vi "CRYMain Menu Process LIB LIB.vi"(9 "sOption":string, 11 "sAction":string) -> (2 "sData_Out":string)   [LabVIEW 2013]
uses:
  CRYProject/CRYProject Editor Global.vi
  CRYMainGlobal.vi
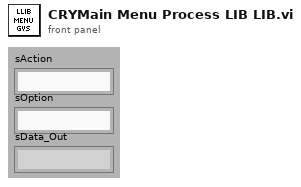
[diagram p1: front panel]
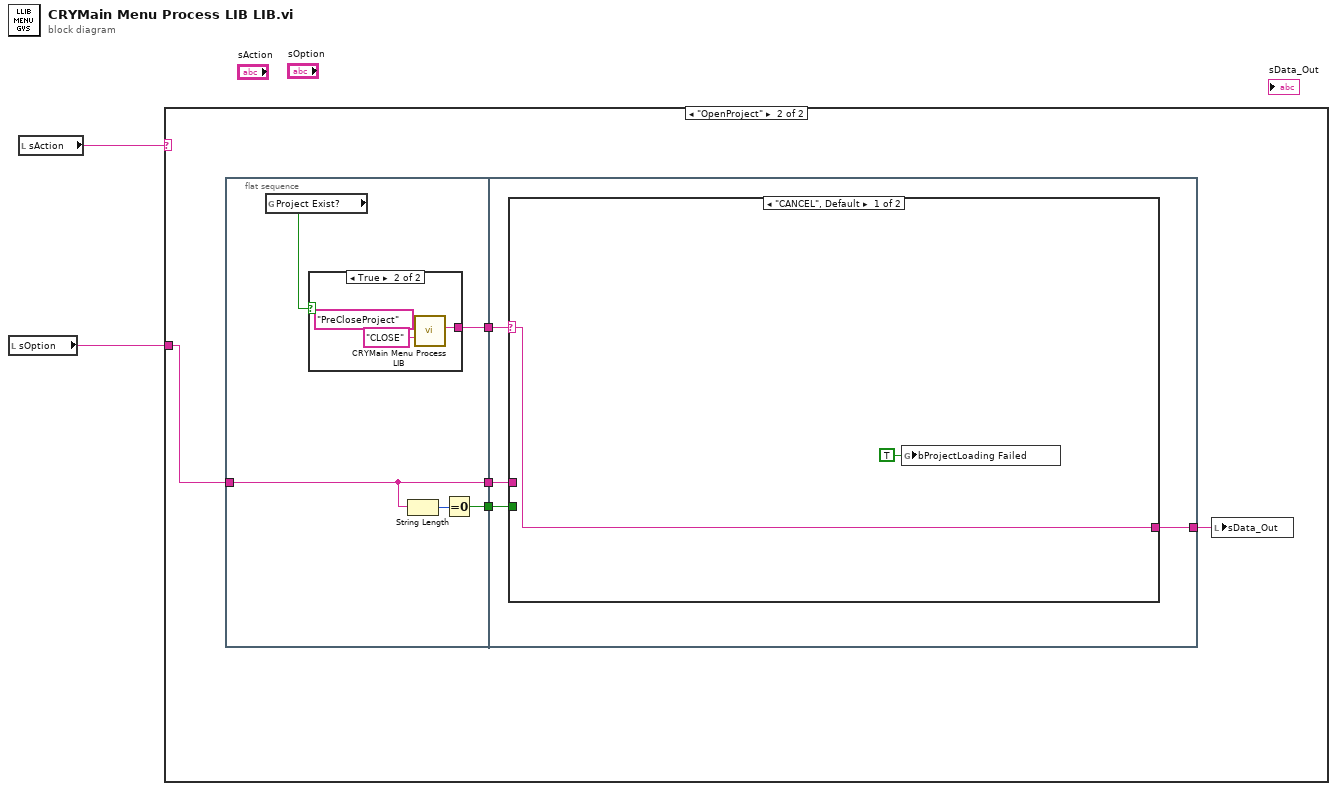
[diagram p0: block diagram]
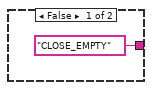
[diagram p3: hidden frame]
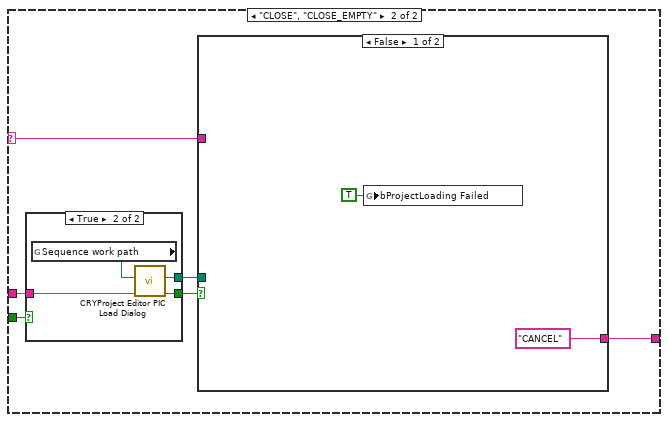
[diagram p4: hidden frame]
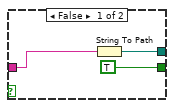
[diagram p5: hidden frame]
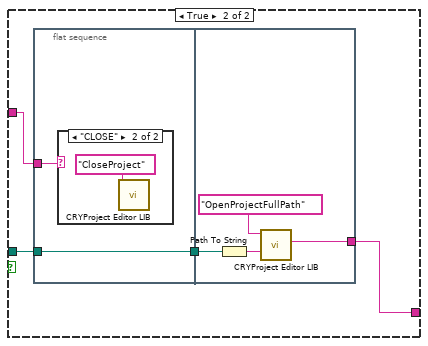
[diagram p6: hidden frame]
diagram:
  n1 = local read "sOption"() -> (w1:string)
  n2 = local read "sAction"() -> (w2:string)
  n3 = case shown="\"OpenProject\"" w2 {
    tunnel: w1 -> [_ w4]
    frame "False", Default {
    }
    frame "OpenProject" {
      n4 = flat-sequence {
        tunnel: [w11] -> w7
        tunnel: [w8] -> w6
        tunnel: [w9] -> w5
        tunnel: w4 -> [w8]
        tunnel: w7 -> [w20]
        tunnel: w6 -> [w19]
        tunnel: w5 -> [w18]
        tunnel: [w17] -> w3
        frame #0 {
          n5 = global read "CRYProject Editor Global.vi" "Project Exist?"() -> (w12:bool)
          n6 = case shown="True" w12 {
            tunnel: ["CLOSE_EMPTY" ("sData_Out") w14] -> w11
            frame False {
            }
            frame True {
              n7 = call "CRYMain Menu Process LIB.vi"("sOption"="CLOSE", "sAction"="PreCloseProject") -> ("sData_Out"=w14:string)  [unwired: 9 in]
            }
          }
          n8 = String Length(string=w8) -> (length=w10:i32)
          n9 = Equal To 0?(x=w10) -> (x = 0?=w9:bool)
        }
        frame #1 {
          n10 = case shown="\"CANCEL\", Default" w20 {
            selector: w20 -> [w22 w26]
            tunnel: w19 -> [_ w25]
            tunnel: w18 -> [_ w24]
            tunnel: [w22 w23] -> w17
            frame "CANCEL", Default {
              n11 = global write "CRYProject Editor Global.vi" "bProjectLoading Failed"(TRUE ("bProjectLoaded Failed")) -> ()
            }
            frame "CLOSE", "CLOSE_EMPTY" {
              n12 = case shown="True" w24 {
                tunnel: [TRUE ("bResult") w34] -> w28
                tunnel: [w30 w33] -> w27
                tunnel: w25 -> [w29 w32]
                frame False {
                  n13 = String To Path(string=w29) -> (path=w30:path)
                }
                frame True {
                  n14 = global read "CRYMainGlobal.vi" "Sequence work path"() -> (w35:path)
                  n15 = call "CRYProject Editor PIC Load Dialog.vi"("File Name"=w32, "Sequence folder path"=w35) -> ("bResult"=w34:bool, "pPathFull"=w33:path)  [unwired: 8 in]
                }
              }
              n16 = case shown="False" w28 {
                tunnel: w27 -> [_ w39]
                tunnel: w26 -> [_ w41]
                tunnel: ["CANCEL" w38] -> w23
                frame False {
                  n17 = global write "CRYProject Editor Global.vi" "bProjectLoading Failed"(TRUE ("bProjectLoaded Failed")) -> ()
                }
                frame True {
                  n18 = flat-sequence {
                    tunnel: w41 -> [w43]
                    tunnel: [w42] -> w40
                    tunnel: w39 -> [w42]
                    tunnel: w40 -> [w46]
                    tunnel: [w45] -> w38
                    frame #0 {
                      n19 = case shown="\"CLOSE\"" w43 {
                        frame Default {
                        }
                        frame "CLOSE" {
                          n20 = call "CRYProject Editor LIB.vi"("sAction"="CloseProject") -> ()  [unwired: 10 in, 1 out]
                        }
                      }
                    }
                    frame #1 {
                      n21 = Path To String(path=w46) -> (string=w47:string)
                      n22 = call "CRYProject Editor LIB.vi"("sData"=w47, "sAction"="OpenProjectFullPath") -> ("sData_Out"=w45:string)  [unwired: 9 in]
                    }
                  }
                }
              }
            }
          }
        }
      }
      n23 = local write "sData_Out"(w3) -> ()
    }
  }
